vi "parse.description.vi"(7 "body":string, 8 "error in (no error)":errorcluster, 11 "issue_class in":refnum<class "issue_class.lvclass">) -> (0 "error out":errorcluster, 3 "issue_class out":refnum<class "issue_class.lvclass">)   [LabVIEW 2024, in "issue_class.lvclass"]
uses:
  issue_class.lvclass
  issue_class.lvclass/issue_class.ctl
  <vilib>/Utility/error.llb/Trim Whitespace.vi
  <vilib>/Utility/error.llb/Trim Whitespace One-Sided.vi
  <userlib>/_OpenG.lib/string/string.llb/openg_string.lvlib
panel:
  out "string out":string
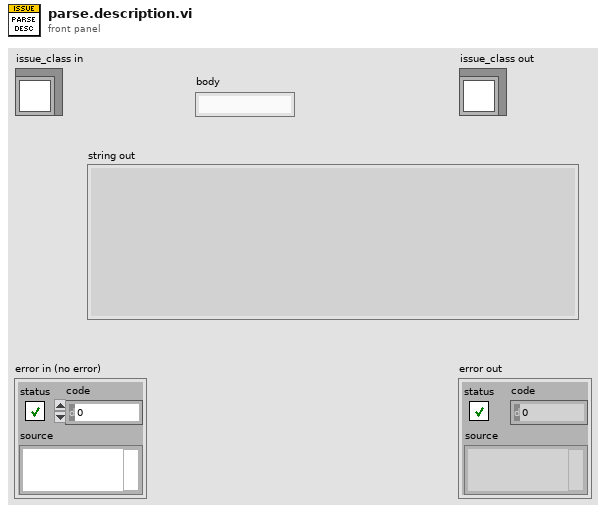
[diagram p1: front panel]
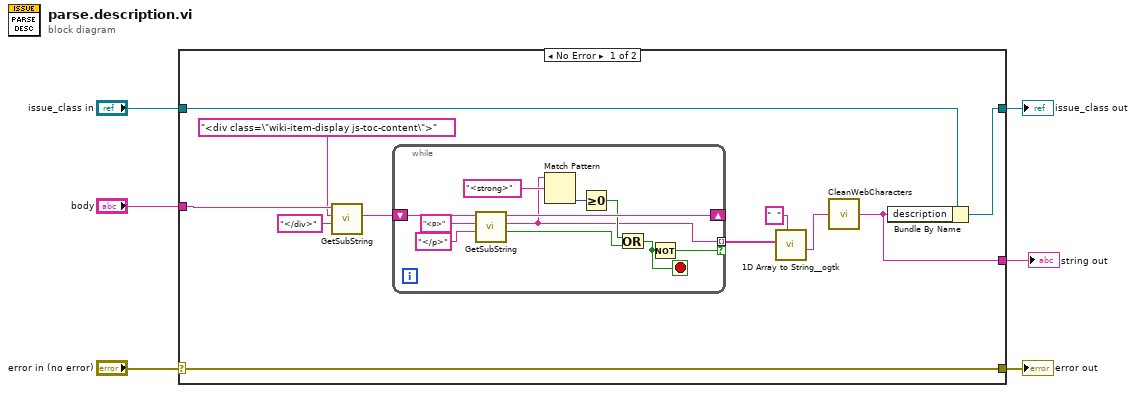
[diagram p0: block diagram]
diagram:
  n1 = case shown="No Error" "error in (no error)" {
    selector: "error in (no error)" -> [w17 w30]
    tunnel: [w17 w30] -> w5
    tunnel: [w15 w29] -> w3
    tunnel: "issue_class in" -> [w16 w29]
    tunnel: "body" -> [w14 _]
    tunnel: [w7 _] -> w1
    frame No Error {
      n2 = call "GetSubString.vi"("End Search"="</div>", "Start Search"="<div class=\"wiki-item-display js-toc-content\">", "String In"=w14) -> ("Match"=w11:string)  [unwired: 6 in, 2 out]
      n3 = while {
        shift-right: [w24] -> _
        shift-left: w11 -> [w28]
        tunnel: [w18] -> w10 mode=indexing if=w25
        stop <- w21 stop-if-true
        n4 = call "GetSubString.vi"("End Search"="</p>", "Start Search"="<p>", "String In"=w28) -> ("Not Found?"=w19:bool, "Match"=w18:string, "Following String Out"=w24:string)  [unwired: 6 in]
        n5 = Match Pattern(string=w18, regular expression="<strong>") -> (offset past match=w22:i32)  [unwired: 1 in, 3 out]
        n6 = Greater Or Equal To 0?(x=w22) -> (x >= 0?=w20:bool)
        n7 = Or(x=w20, y=w19) -> (x .or. y?=w21:bool)
        n8 = Not(x=w21) -> (.not. x?=w25:bool)
      }
      n9 = call <userlib>:"1D Array to String__ogtk.vi"("delimiter (Tab)"="  ", "Array of Strings"=w10) -> ("delimited string"=w8:string)  [unwired: 9 in]
      n10 = call "CleanWebCharacters.vi"("string in"=w8) -> ("string out"=w7:string)
      n11 = Bundle By Name(cluster=w16, "description"=w7) -> (w15:refnum<class "issue_class.lvclass">)
    }
    frame Error {
    }
  }
  "error out" <- w5
  "issue_class out" <- w3
  "string out" <- w1
